vi "FRCts20_WebMethods_Competition_DELETE.vi"(7 "httpRequestID":u32, 11 "competition":string) -> ()   [LabVIEW 2014]
doc: "<B>DELETE</B> the specified <B>competition</B> resource\n\nhttp://<server address>:<port>/FRCts/competition/<B>competition</B>\n\n{requires authentication}"
uses:
  FRCts20_WebMethods.lvlib
  <vilib>/wsapi/NI_WebServices.lvlib
  Backend/source/VI Source/FRCts20_Backend_API/FRCts20_Backend_API.lvlib
  Backend/source/VI Source/FRCts20_Backend_API/FRCts20_Backend_API_Competition.ctl
  Backend/source/VI Source/FRCts20_Backend_API/FRCts20_Backend_API_Command_Competition.ctl
  Backend/source/VI Source/FRCts20_Backend_API/FRCts20_Backend_API_Comment.vi
panel:
  in  "query":string
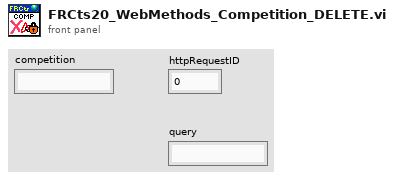
[diagram p1: front panel]
types:
  T1 = typedef "FRCts20_Backend_API.lvlib/FRCts20_Backend_API_Command_Competition.ctl" = string
  T2 = typedef "FRCts20_Backend_API.lvlib/FRCts20_Backend_API_Competition.ctl" = cluster{"Name":string, "Start Date":timestamp, "Duration":u8, "Divisions":string[], "APIReturn":string}
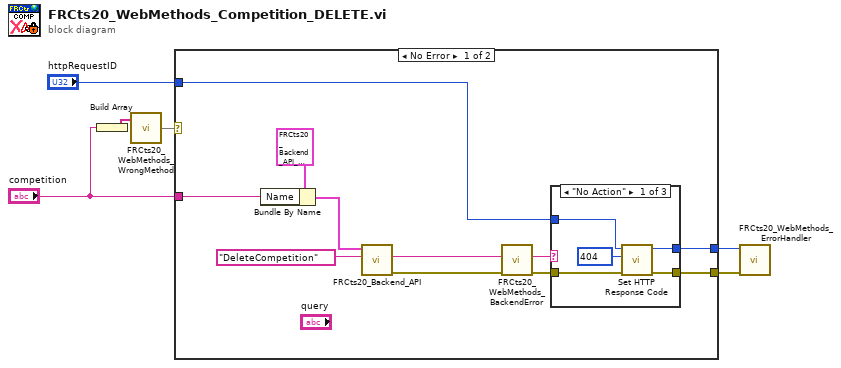
[diagram p0: block diagram]
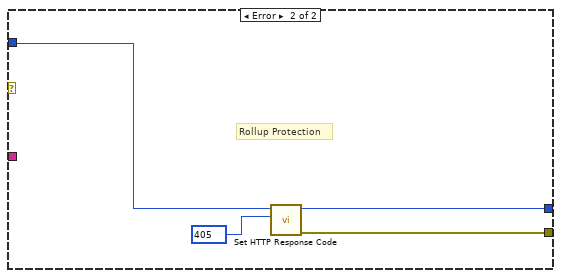
[diagram p4: hidden frame]
diagram:
  n1 = Build Array("competition") -> (w2:string[])
  n2 = call "FRCts20_WebMethods_WrongMethod.vi"(4:w2) -> (1:w3)  [unwired: 3 in, 1 out]
  n3 = case shown="No Error" w3 {
    tunnel: "httpRequestID" -> [w11 w27]
    tunnel: [w13 w29] -> w5
    tunnel: [w12 w28] -> w4
    tunnel: "competition" -> [w9 _]
    frame No Error {
      n4 = Bundle By Name(cluster=T2 {"Name"="", "Start Date"=timestamp(0 s since 1904-01-01), "Duration"=0, "Divisions"=[], "APIReturn"=""} ("Competition"), "Name"=w9) -> (w8:T2)
      n5 = call-poly "FRCts20_Backend_API.vi"("Command"=T1 "DeleteCompetition", "Note In"=w8) -> ("error out"=w17:errorcluster, "Status"=w16:string)  [unwired: 7 in, 1 out]
      n6 = call "FRCts20_WebMethods_BackendError.vi"("error in (no error)"=w17, "Status"=w16) -> ("error out"=w14:errorcluster, "Status out"=w15:string)  [unwired: 8 in]
      n7 = case shown="\"No Action\"" w15 {
        tunnel: w14 -> [w19 w24 w26]
        tunnel: [w22 w24 w26] -> w13
        tunnel: w11 -> [w20 w23 w25]
        tunnel: [w21 w23 w25] -> w12
        frame "No Action" {
          w18 = 404 items=["100"=100, "101"=101, "200"=200, "201"=201, "202"=202, "203"=203, "204"=204, "205"=205, "206"=206, "300"=300, "301"=301, "302"=302, "303"=303, "304"=304, "305"=305, "306"=306, "307"=307, "400"=400, "401"=401, "402"=402, "403"=403, "404"=404, "405"=405, "406"=406, "407"=407, "408"=408, "409"=409, "410"=410, "411"=411, "412"=412, "413"=413, "414"=414, "415"=415, "416"=416, "417"=417, "500"=500, "501"=501, "502"=502, "503"=503, "504"=504, "505"=505] ("response code (200)")
          n8 = call <vilib>:"Set HTTP Response Code.vi"("error in (no error)"=w19, "response code (200)"=w18, "httpRequestID"=w20) -> ("error out"=w22:errorcluster, "httpRequestID out"=w21:u32)  [unwired: 7 in]
        }
        frame "Backend Error", Default {
        }
        frame "Success" {
        }
      }
    }
    frame Error {
      w30 = 405 items=["100"=100, "101"=101, "200"=200, "201"=201, "202"=202, "203"=203, "204"=204, "205"=205, "206"=206, "300"=300, "301"=301, "302"=302, "303"=303, "304"=304, "305"=305, "306"=306, "307"=307, "400"=400, "401"=401, "402"=402, "403"=403, "404"=404, "405"=405, "406"=406, "407"=407, "408"=408, "409"=409, "410"=410, "411"=411, "412"=412, "413"=413, "414"=414, "415"=415, "416"=416, "417"=417, "500"=500, "501"=501, "502"=502, "503"=503, "504"=504, "505"=505] ("response code (200)")
      # "Rollup Protection"
      n9 = call <vilib>:"Set HTTP Response Code.vi"("response code (200)"=w30, "httpRequestID"=w27) -> ("error out"=w29:errorcluster, "httpRequestID out"=w28:u32)  [unwired: 8 in]
    }
  }
  n10 = call "FRCts20_WebMethods_ErrorHandler.vi"("error in"=w5, "httpRequestID"=w4) -> ()  [unwired: 9 in, 1 out]
